vi "filter.test.Delete.Only.Order.vi"() -> ()   [LabVIEW 2020]
uses:
  Market.Data.Common/host/fpganow.common.host.lvlib
  Market.Data.Common/fpga/orderbook.command.ctl
  Market.Data.Common/fpga/fpganow.common.fpga.lvlib
  Market.Data.Common/fpga/orderbook.command.type.ctl
panel:
  out "error out":errorcluster
  out "GetState":u64[](array[numeric]) format="%.0x"
  in  "Expected.GetState":u64[](array[numeric])=[4702127773838221344, 176, 6076284164848492576, 177] format="%.0x"
  out "Debug":u64[](array[numeric]) format="%.0x"
  out "Passed":bool
  out "OrderBook.Commands.out":T1[](array[typedef]) {"symbol" format="%.0x"; "orderId" format="%.0x"; "side" format="%.0x"}
  in  "OrderBook.Commands.in":T1[](array[typedef])=[{"type"=enum."AddOrder", "side"=66, "orderId "=48, "quantity"=100, "symbol"=4702127773838221344, "price"=9050, "executed.qty"=0, "canceled.qty"=0, "remaining.qty"=0, "seconds"=0, "nanoseconds"=0, "Add"=TRUE, "Edit"=FALSE, "Remove"=FALSE, "seq no"=1, "recv.time"=0, "parse.time"=0}, {"type"=enum."OrderExecuted", "side"=66, "orderId "=48, "quantity"=0, "symbol"=0, "price"=9050, "executed.qty"=100, "canceled.qty"=0, "remaining.qty"=0, "seconds"=0, "nanoseconds"=0, "Add"=FALSE, "Edit"=FALSE, "Remove"=FALSE, "seq no"=2, "recv.time"=0, "parse.time"=0}] {"symbol" format="%.0x"; "quantity" format="%.0x"; "orderId" format="%.0x"; "side" format="%.0x"}
  in  "Watch.List":string[](array[string])=["AAPL", "TSLA"]
  in  "Expected OrderBook.Commands":T1[](array[typedef])=[{"type"=enum."AddOrder", "side"=66, "orderId "=48, "quantity"=100, "symbol"=4702127773838221344, "price"=9050, "executed.qty"=0, "canceled.qty"=0, "remaining.qty"=0, "seconds"=0, "nanoseconds"=0, "Add"=TRUE, "Edit"=FALSE, "Remove"=FALSE, "seq no"=1, "recv.time"=0, "parse.time"=0}, {"type"=enum."OrderExecuted", "side"=66, "orderId "=48, "quantity"=0, "symbol"=0, "price"=9050, "executed.qty"=100, "canceled.qty"=0, "remaining.qty"=0, "seconds"=0, "nanoseconds"=0, "Add"=FALSE, "Edit"=FALSE, "Remove"=FALSE, "seq no"=2, "recv.time"=0, "parse.time"=0}] {"symbol" format="%.0x"; "orderId" format="%.0x"; "side" format="%.0x"}
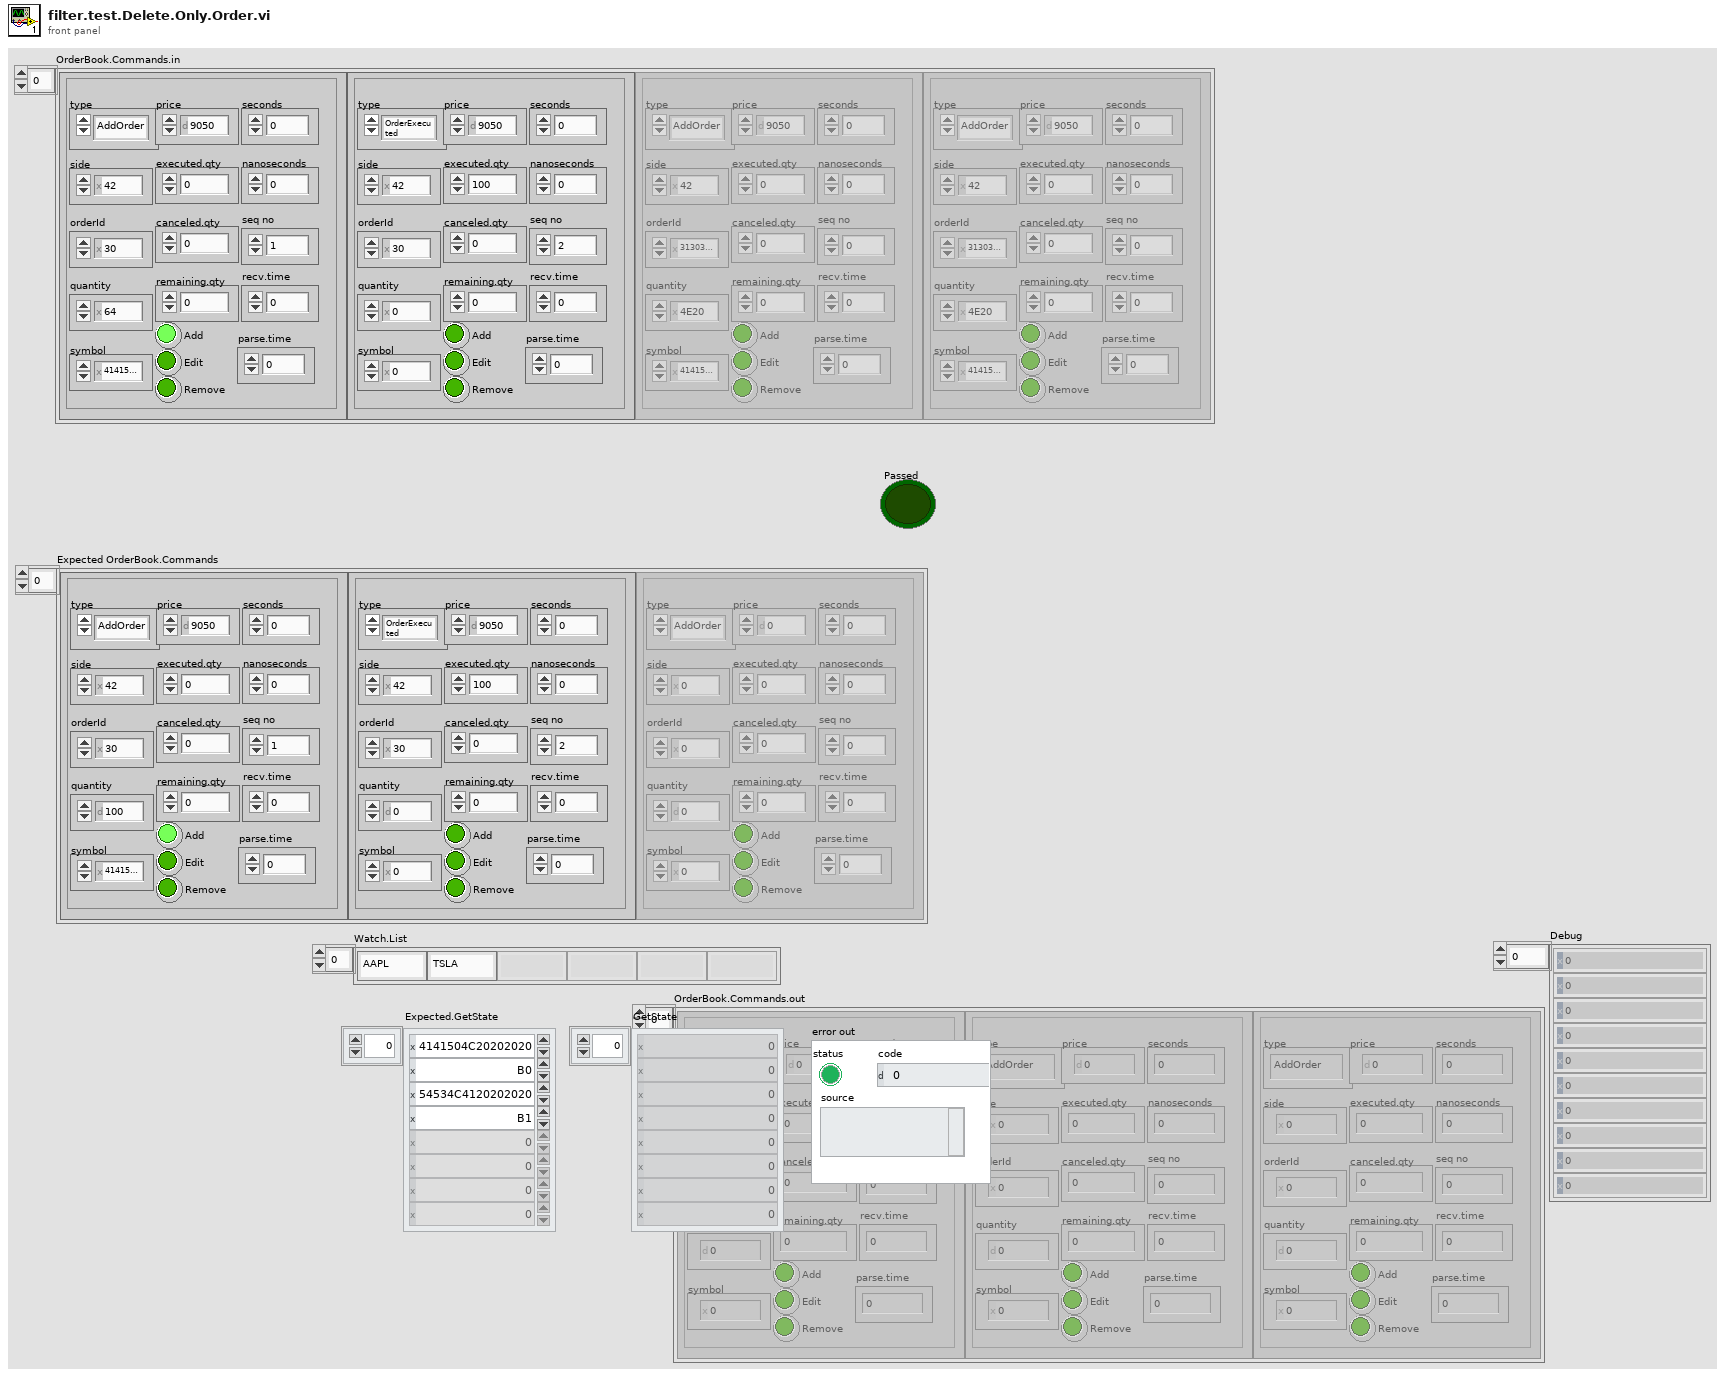
[diagram p1: front panel]
types:
  T1 = typedef "fpganow.common.fpga.lvlib/orderbook.command.ctl" = cluster{"type":T2, "side":u8, "orderId ":u64, "quantity":u32, "symbol":u64, "price":u64, "executed.qty":u32, "canceled.qty":u32, "remaining.qty":u32, "seconds":u64, "nanoseconds":u64, "Add":bool, "Edit":bool, "Remove":bool, "seq no":u32, "recv.time":u64, "parse.time":u64}
  T2 = typedef "fpganow.common.fpga.lvlib/orderbook.command.type.ctl" = enum8{"Time", "AddOrder", "OrderExecuted", "OrderExecutedAtPrice", "ReduceSize", "ModifyOrder", "DeleteOrder", "Get.Everything", "Get.All.Orders", "Get.Top"}
  T3 = cluster{"Match.Defaults":bool[][], "Failures.Count":i32, "Passed":bool}
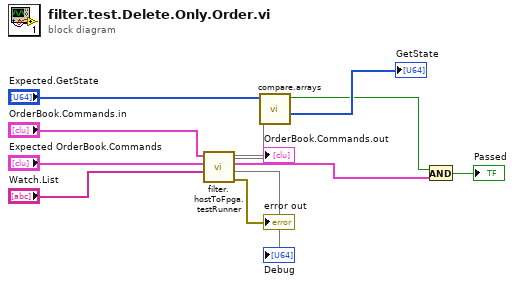
[diagram p0: block diagram]
diagram:
  n1 = call "filter.hostToFpga.testRunner.vi"("Watch.List"="Watch.List", "Expected OrderBook.Command[]"="Expected OrderBook.Commands", "OrderBook.Commands.in"="OrderBook.Commands.in") -> ("error out"=→"error out":errorcluster, "Metadata.Results.out"=w2:T3, 3:→"OrderBook.Commands.out", 4:→"Debug", 5:w6)  [unwired: 3 in, 1 out]
  n2 = call "compare.arrays.vi"("Actual"=w6, "Expected"="Expected.GetState") -> ("Actual.Out"=→"GetState":u64[], "Full.Match"=w3:bool)  [unwired: 7 in, 1 out]
  n3 = And(x=w3, y=w2) -> (x .and. y?=→"Passed":bool)
